vi "VI Tester Plugin - Plugin -.vi"(8 "error in":errorcluster) -> (0 "error out":errorcluster)   [LabVIEW 2009]
uses:
  <vilib>/addons/_JKI Toolkits/RCF API/Right Click API.llb/Right Click API Plugin Info Data__RightClickAPI.ctl
  <vilib>/picture/picture.llb/imagedata.ctl
  <vilib>/addons/_JKI Toolkits/RCF API/Right Click API.llb/Right Click API Menu Activation Data__RightClickAPI.ctl
  <vilib>/addons/_JKI Toolkits/RCF API/Right Click API.llb/Generic Option - Input Data - __RightClickAPI.ctl
  <vilib>/addons/_JKI Toolkits/RCF API/Right Click API.llb/RightClickAPI.lvlib
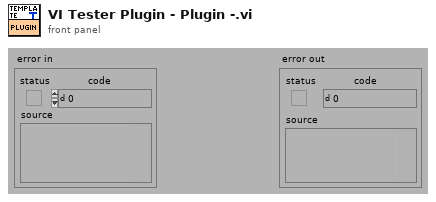
[diagram p1: front panel]
types:
  T1 = cluster{"Last Test":string, "Recent Tests":string}
  T2 = typedef "imagedata.ctl" = cluster{"image type":i32, "image depth":i32, "image":u8[], "mask":u8[], "colors":u32[], "Rectangle":cluster{"left":i16, "top":i16, "right":i16, "bottom":i16}}
  T3 = typedef "RightClickAPI.lvlib/Right Click API Plugin Info Data__RightClickAPI.ctl" = cluster{"Name":string, "Summary":string, "Description":string, "Copyright":string, "License":string, "Developer":string, "Version":string, "Plugin Glyph (32x32)":T2}
  T4 = typedef "RightClickAPI.lvlib/Right Click API Framework Data__RightClickAPI.ctl" = cluster{"Active VI Info":T5, "Mode":T7, "Shortcut Menu Selection":T8, "Plugins Options":T9}
  T5 = typedef "RightClickAPI.lvlib/Framework - Active VI Info - Cluster - __RightClickAPI.ctl" = cluster{"Active VI Refnum":refnum<vi>, "Active VI Type":T6, "Active VI Sel. List[]":refnum<vi>[], "Mouse Coords":cluster{"Horizontal":i32, "Vertical":i32}}
  T6 = typedef "RightClickAPI.lvlib/Framework - Selection Type - Enum - __RightClickAPI.ctl" = enum16{"Panel", "Diagram"}
  T7 = typedef "RightClickAPI.lvlib/Right Click API - Mode - Enum - __RightClickAPI.ctl" = enum16{"Initialize", "Menu Activation", "Menu Selection", "Edit Options"}
  T8 = typedef "RightClickAPI.lvlib/Framework - Shortcut Menu Selection Events - Cluster - __RightClickAPI.ctl" = cluster{"ItemTag":string, "ItemPath":string, "Coords":cluster{"Horizontal":i32, "Vertical":i32}}
  T9 = typedef "RightClickAPI.lvlib/Framework - Plugin Options - Cluster - __RightClickAPI.ctl" = cluster{"Config Data":string}
  T10 = typedef "RightClickAPI.lvlib/Right Click API Menu Activation Data__RightClickAPI.ctl" = cluster{"Menu String":string}
  T11 = typedef "RightClickAPI.lvlib/Generic Option - Input Data - __RightClickAPI.ctl" = cluster{"Config Data":variant}
  T12 = typedef "RightClickAPI.lvlib/Generic Option - Output Data - __RightClickAPI.ctl" = cluster{"Config Data":variant}
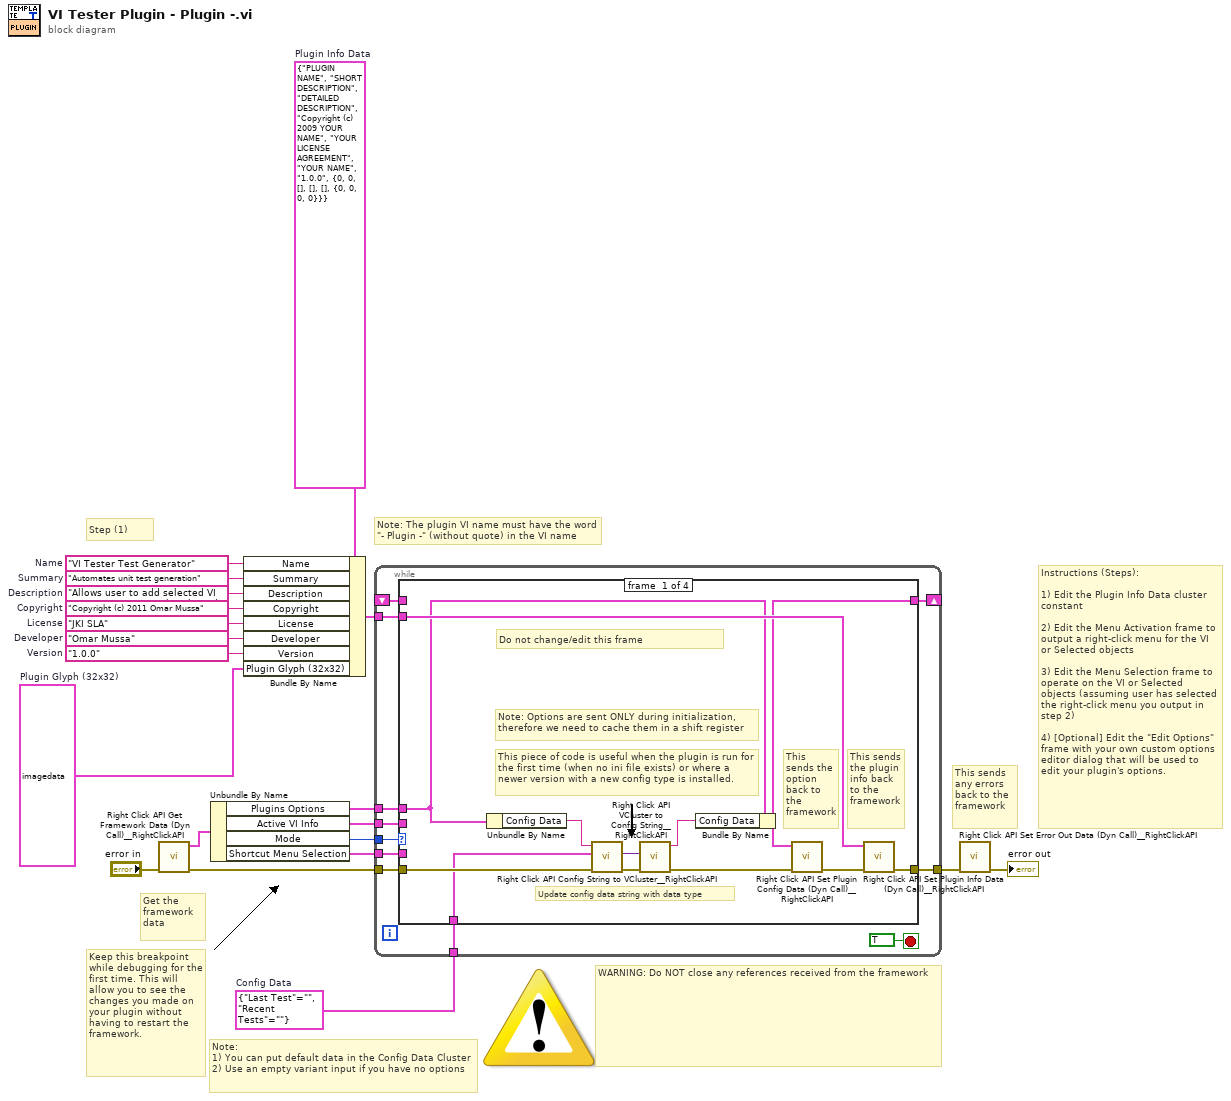
[diagram p0: block diagram]
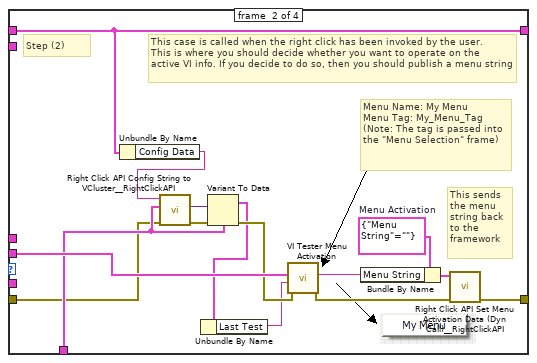
[diagram p2: hidden frame]
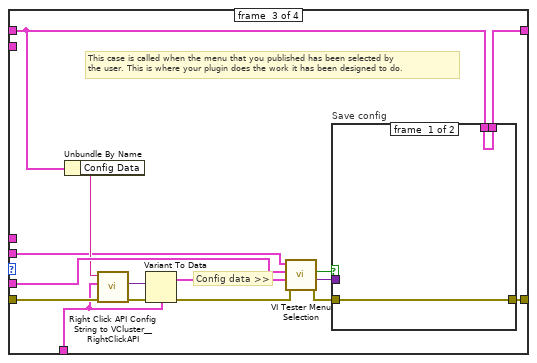
[diagram p3: hidden frame]
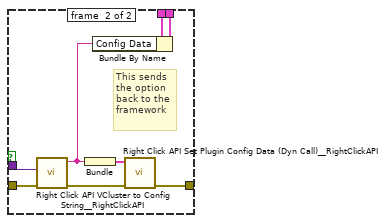
[diagram p4: hidden frame]
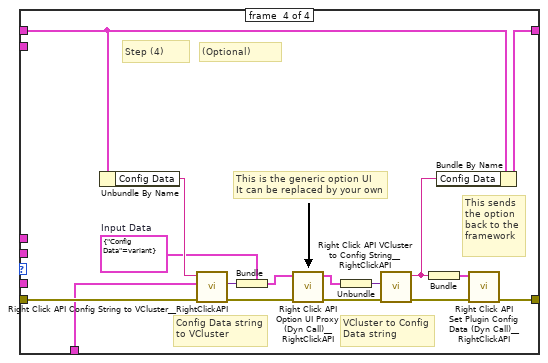
[diagram p5: hidden frame]
diagram:
  w11 = T1 {"Last Test"="", "Recent Tests"=""}  # Config Data
  w1 = T2 {"image type"=0, "image depth"=32, "image"=array[4096 elements], "mask"=[0, 0, 0, 0, 0, 0, 0, 0, 0, 4, 0, 0, 0, 31, 0, 0, 126, 31, 0, 0, 127, 31, 0, 0, 127, 159, 0, 0, 127, 196, 0, 0, 127, 192, 0, 0, 127, 221, 155, 182, 127, 201, 33, 37, 127, 201, 145, 54, 127, 201, 9, 37, 127, 201, 177, 53, 127, 224, 0, 0, 127, 224, 0, 0, 15, 224, 0, 0, 15, 224, 0, 0, 15, 224, 0, 0, 15, 224, 0, 0, 15, 224, 0, 0, 15, 224, 0, 0, 0, 0, 0, 0, 0, 0, 0, 0, 0, 0, 0, 0, 0, 0, 0, 0, 0, 0, 0, 0, 0, 0, 0, 0, 0, 0, 0, 0, 0, 0, 0, 0, 0, 0, 0, 0, 0, 0, 0, 0], "colors"=[], "Rectangle"={"left"=0, "top"=0, "right"=32, "bottom"=32}}  # Plugin Glyph (32x32)
  w2 = "1.0.0"  # Version
  w3 = "Omar Mussa"  # Developer
  w4 = "JKI SLA"  # License
  w5 = "Copyright (c) 2011 Omar Mussa"  # Copyright
  w6 = "Allows user to add selected VI to a new or previously selected test."  # Description
  w7 = "Automates unit test generation"  # Summary
  w8 = "VI Tester Test Generator"  # Name
  w9 = T3 {"Name"="PLUGIN NAME", "Summary"="SHORT DESCRIPTION", "Description"="DETAILED DESCRIPTION", "Copyright"="Copyright (c) 2009 YOUR NAME", "License"="YOUR LICENSE AGREEMENT", "Developer"="YOUR NAME", "Version"="1.0.0", "Plugin Glyph (32x32)"={"image type"=0, "image depth"=0, "image"=[], "mask"=[], "colors"=[], "Rectangle"={"left"=0, "top"=0, "right"=0, "bottom"=0}}}  # Plugin Info Data
  # "Keep this breakpoint while debugging for the first time. This will allow you to see the changes you made on your plugin without having to restart the framework."
  # "WARNING: Do NOT close any references received from the framework"
  # "Step (1)"
  # "Instructions (Steps):\n\n1) Edit the Plugin Info Data cluster constant\n\n2) Edit the Menu Activation frame to output a right-click menu for the VI or Selected objects\n\n3) Edit the Menu Selection frame to operate on the VI or Selected objects (assuming user has selected the right-click menu you output in step 2)\n\n4) [Optional] Edit the \"Edit Options\" frame with your own custom options editor dialog that will be used to edit your plugin's options."
  # "Note: The plugin VI name must have the word \n\"- Plugin -\" (without quote) in the VI name"
  # "Get the framework data"
  # "This sends any errors back to the framework"
  # "Note:\n1) You can put default data in the Config Data Cluster\n2) Use an empty variant input if you have no options"
  n1 = call <vilib>:"Right Click API Get Framework Data (Dyn Call)__RightClickAPI.vi"("error in (no error)"="error in") -> ("error out"=w14:errorcluster, "Framework Data"=w13:T4)  [unwired: 9 in]
  n2 = Unbundle By Name(w13) -> ("Plugins Options"=w12:T9, "Active VI Info"=w19:T5, "Mode"=w20:T7, "Shortcut Menu Selection"=w18:T8)
  n3 = Bundle By Name(cluster=w9, "Name"=w8, "Summary"=w7, "Description"=w6, "Copyright"=w5, "License"=w4, "Developer"=w3, "Version"=w2, "Plugin Glyph (32x32)"=w1) -> (w10:T3)
  n4 = while {
    tunnel: w20 -> [w31]
    tunnel: w19 -> [w30]
    tunnel: w18 -> [w29]
    tunnel: [w28] -> w17
    tunnel: w14 -> [w27]
    tunnel: w10 -> [w26]
    shift-right: [w23] -> _
    shift-left: _ -> [w22]
    tunnel: w12 -> [w24]
    tunnel: w11 -> [w21]
    stop <- TRUE stop-if-true
    n5 = case shown="\"Initialize\"" w31 {
      tunnel: w27 -> [w40 w49 w71 w97]
      tunnel: [w43 w58 w62 w91] -> w28
      tunnel: w30 -> [_ w53 w67 _]
      tunnel: w29 -> [_ _ w73 _]
      tunnel: w26 -> [w42 _ _ _]
      tunnel: w24 -> [w35 _ _ _]
      tunnel: [w32 w52 w60 w98] -> w23
      tunnel: w22 -> [_ w52 w61 w99]
      tunnel: w21 -> [w38 w50 w69 w96]
      frame #0 {
        # "Do not change/edit this frame"
        # "Update config data string with data type"
        # "This sends the plugin info back to the framework"
        # "This sends the option back to the framework"
        # "This piece of code is useful when the plugin is run for the first time (when no ini file exists) or where a newer version with a new config type is installed."
        # "Note: Options are sent ONLY during initialization, therefore we need to cache them in a shift register"
        n6 = Unbundle By Name(w35) -> ("Config Data"=w37:string)
        n7 = call <vilib>:"Right Click API Config String to VCluster__RightClickAPI.vi"("error in (no error)"=w40, "type"=w38, "Config String"=w37) -> ("error out"=w41:errorcluster, "VCluster"=w39:variant)  [unwired: 7 in]
        n8 = call <vilib>:"Right Click API VCluster to Config String__RightClickAPI.vi"("error in (no error)"=w41, "VCluster"=w39) -> ("error out"=w33:errorcluster, "Config String"=w36:string)  [unwired: 8 in]
        n9 = Bundle By Name(cluster=w35, "Config Data"=w36) -> (w32:T9)
        n10 = call <vilib>:"Right Click API Set Plugin Config Data (Dyn Call)__RightClickAPI.vi"("error in (no error)"=w33, "Plugins Options"=w32) -> ("error out"=w34:errorcluster)  [unwired: 9 in]
        n11 = call <vilib>:"Right Click API Set Plugin Info Data (Dyn Call)__RightClickAPI.vi"("error in (no error)"=w34, "Plugin Info Data"=w42) -> ("error out"=w43:errorcluster)  [unwired: 9 in]
      }
      frame #1 {
        w54 = T10 {"Menu String"=""}  # Menu Activation
        # "Menu Name: My Menu\nMenu Tag: My_Menu_Tag\n(Note: The tag is passed into the \"Menu Selection\" frame)"
        # "Step (2)"
        # "This sends the menu string back to the framework"
        # "This case is called when the right click has been invoked by the user.\nThis is where you should decide whether you want to operate on the \nactive VI info. If you decide to do so, then you should publish a menu string"
        n12 = Unbundle By Name(w52) -> ("Config Data"=w51:string)
        n13 = call <vilib>:"Right Click API Config String to VCluster__RightClickAPI.vi"("error in (no error)"=w49, "type"=w50, "Config String"=w51) -> ("error out"=w47:errorcluster, "VCluster"=w46:variant)  [unwired: 7 in]
        n14 = Variant To Data(error in=w47, Variant=w46, type=w50) -> (error out=w48:errorcluster, data=w45:T1)
        n15 = Unbundle By Name(w45) -> ("Last Test"=w44:string)
        n16 = call "VI Tester Menu Activation.vi"("error in"=w48, "Last Test"=w44, "Active VI Info"=w53) -> ("error out"=w57:errorcluster, "Menu String"=w56:string)  [unwired: 7 in]
        n17 = Bundle By Name(cluster=w54, "Menu String"=w56) -> (w55:T10)
        n18 = call <vilib>:"Right Click API Set Menu Activation Data (Dyn Call)__RightClickAPI.vi"("error in (no error)"=w57, "Menu Activation Data"=w55) -> ("error out"=w58:errorcluster)  [unwired: 9 in]
      }
      frame #2 {
        # "Config data >>"
        # "This case is called when the menu that you published has been selected by\nthe user. This is where your plugin does the work it has been designed to do."
        n19 = Unbundle By Name(w61) -> ("Config Data"=w70:string)
        n20 = call <vilib>:"Right Click API Config String to VCluster__RightClickAPI.vi"("error in (no error)"=w71, "type"=w69, "Config String"=w70) -> ("error out"=w66:errorcluster, "VCluster"=w65:variant)  [unwired: 7 in]
        n21 = Variant To Data(error in=w66, Variant=w65, type=w69) -> (error out=w72:errorcluster, data=w68:T1)
        n22 = call "VI Tester Menu Selection.vi"("error in"=w72, "Config In"=w68, "Shortcut Menu Selection"=w73, "Active VI Info"=w67) -> ("error out"=w63:errorcluster, "Config Out"=w64:variant, "Config Changed"=w59:bool)  [unwired: 5 in]
        n23 = case "Save config" shown="True" w59 {
          tunnel: w64 -> [_ w80]
          tunnel: w63 -> [w74 w79]
          tunnel: [w74 w78] -> w62
          tunnel: w61 -> [w75 w77]
          tunnel: [w75 w76] -> w60
          frame #0 {
          }
          frame #1 {
            # "This sends the option back to the framework"
            n24 = call <vilib>:"Right Click API VCluster to Config String__RightClickAPI.vi"("error in (no error)"=w79, "VCluster"=w80) -> ("error out"=w83:errorcluster, "Config String"=w82:string)  [unwired: 8 in]
            n25 = Bundle("Config String"=w82) -> (w81:cluster{"Config String":string})  [unwired: 1 in]
            n26 = Bundle By Name(cluster=w77, "Config Data"=w82) -> (w76:T9)
            n27 = call <vilib>:"Right Click API Set Plugin Config Data (Dyn Call)__RightClickAPI.vi"("error in (no error)"=w83, "Plugins Options"=w81) -> ("error out"=w78:errorcluster)  [unwired: 9 in]
          }
        }
      }
      frame #3 {
        w88 = T11 {"Config Data"=variant}  # Input Data
        # "Step (4)"
        # "(Optional)"
        # "VCluster to Config Data string"
        # "Config Data string to VCluster"
        # "This sends the option back to the framework"
        # "This is the generic option UI\nIt can be replaced by your own"
        n28 = Unbundle By Name(w99) -> ("Config Data"=w95:string)
        n29 = call <vilib>:"Right Click API Config String to VCluster__RightClickAPI.vi"("error in (no error)"=w97, "type"=w96, "Config String"=w95) -> ("error out"=w94:errorcluster, "VCluster"=w87:variant)  [unwired: 7 in]
        n30 = Bundle(cluster=w88, "Config Data"=w87) -> (w86:T11)
        n31 = call <vilib>:"Right Click API Option UI Proxy (Dyn Call)__RightClickAPI.vi"("error in (no error)"=w94, "Input Data"=w86) -> ("error out"=w93:errorcluster, "Output Data"=w85:T12)  [unwired: 8 in]
        n32 = Unbundle(w85) -> ("Config Data"=w84:variant)
        n33 = call <vilib>:"Right Click API VCluster to Config String__RightClickAPI.vi"("error in (no error)"=w93, "VCluster"=w84) -> ("error out"=w92:errorcluster, "Config String"=w90:string)  [unwired: 8 in]
        n34 = Bundle("Config String"=w90) -> (w89:cluster{"Config String":string})  [unwired: 1 in]
        n35 = Bundle By Name(cluster=w99, "Config Data"=w90) -> (w98:T9)
        n36 = call <vilib>:"Right Click API Set Plugin Config Data (Dyn Call)__RightClickAPI.vi"("error in (no error)"=w92, "Plugins Options"=w89) -> ("error out"=w91:errorcluster)  [unwired: 9 in]
      }
    }
  }
  n37 = call <vilib>:"Right Click API Set Error Out Data (Dyn Call)__RightClickAPI.vi"("error in (no error)"=w17) -> ("error out"=→"error out":errorcluster)  [unwired: 10 in]
